vi "pharosSet.vi"(0 "triggers":u8[](array[numeric])) -> ()   [LabVIEW 2017]
uses:
  <vilib>/DAQmx/write.llb/DAQmx Write (Digital 1D U8 1Chan NSamp).vi
  globalDevices.vi
  <vilib>/DAQmx/miscellaneous.llb/DAQmx Fill In Error Info.vi
  globalUtilities.vi
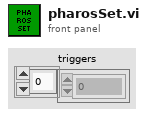
[diagram p1: front panel]
types:
  T1 = enum16{"open", "replace", "create", "open or create", "replace or create", "replace or create with confirmation"}
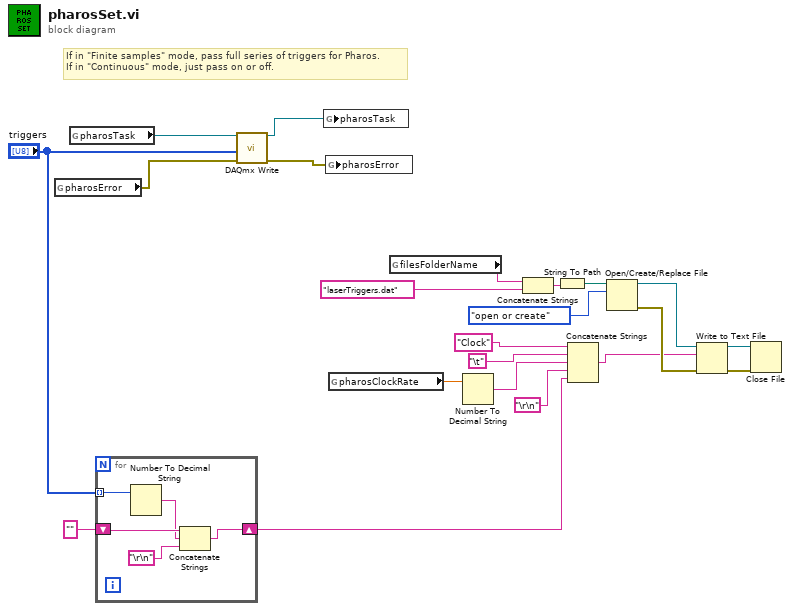
[diagram p0: block diagram]
diagram:
  # "If in \"Finite samples\" mode, pass full series of triggers for Pharos.\nIf in \"Continuous\" mode, just pass on or off."
  n1 = global read "globalDevices.vi" "pharosError"() -> (w21:errorcluster)
  n2 = global read "globalDevices.vi" "pharosTask"() -> (w22:refnum<k21>)
  n3 = for {
    tunnel: "triggers" -> [w25] mode=indexing
    shift-right: [w24] -> w7
    shift-left: "" -> [w27]
    n4 = Number To Decimal String(number=w25) -> (decimal integer string=w26:string)  [unwired: 1 in]
    n5 = Concatenate Strings(w27, w26, "\r\n") -> (w24:string)
  }
  n6 = call-poly <vilib>:"DAQmx Write.vi"("task/channels in"=w22, "data"="triggers", "error in"=w21) -> ("task out"=w20:refnum<k21>, "error out"=w19:errorcluster)  [unwired: 10 in, 1 out]
  n7 = global write "globalDevices.vi" "pharosTask"(w20) -> ()
  n8 = global write "globalDevices.vi" "pharosError"(w19) -> ()
  n9 = global read "globalDevices.vi" "pharosClockRate"() -> (w11:dbl)
  n10 = global read "globalUtilities.vi" "filesFolderName"() -> (w18:string)
  n11 = Number To Decimal String(number=w11) -> (decimal integer string=w10:string)  [unwired: 1 in]
  n12 = Concatenate Strings(w18, "laserTriggers.dat") -> (w16:string)
  n13 = String To Path(string=w16) -> (path=w15:path)
  n14 = Concatenate Strings("Clock", "\t", w10, "\r\n", w7) -> (w6:string)
  n15 = Open/Create/Replace File(file path (use dialog)=w15, operation (0:open)=T1."open or create") -> (refnum out=w13:refnum<file>, error out=w12:errorcluster)  [unwired: 4 in, 1 out]
  n16 = Write to Text File(file (use dialog)=w13, text=w6, error in=w12) -> (refnum out=w4:refnum<file>, error out=w5:errorcluster)  [unwired: 1 in, 1 out]
  n17 = Close File(refnum=w4, error in=w5) -> ()  [unwired: 2 out]
